vi "Threshold.vi"(8 "error in (no error)":errorcluster, 10 "Threshold":dbl, 11 "DAQ AI in":refnum<class "DAQ AI.lvclass">) -> (0 "error out":errorcluster, 3 "DAQ AI out":refnum<class "DAQ AI.lvclass">)   [LabVIEW 2020, in "DAQ AI.lvlib" / "DAQ AI.lvclass"]
uses:
  DAQ AI.lvclass
  DAQ AI.lvclass/DAQ AI.ctl
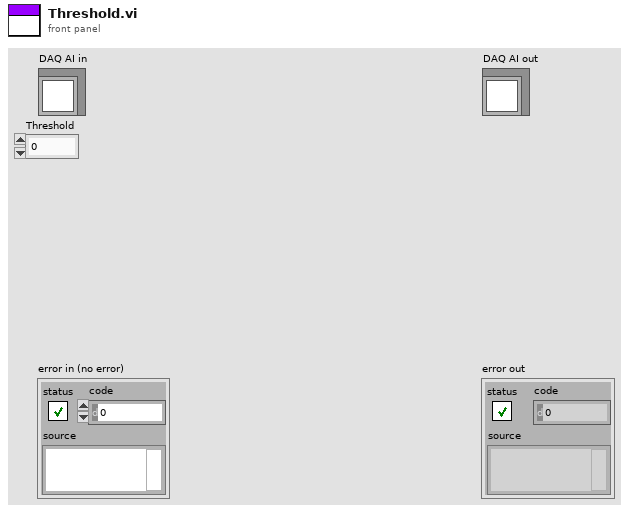
[diagram p1: front panel]
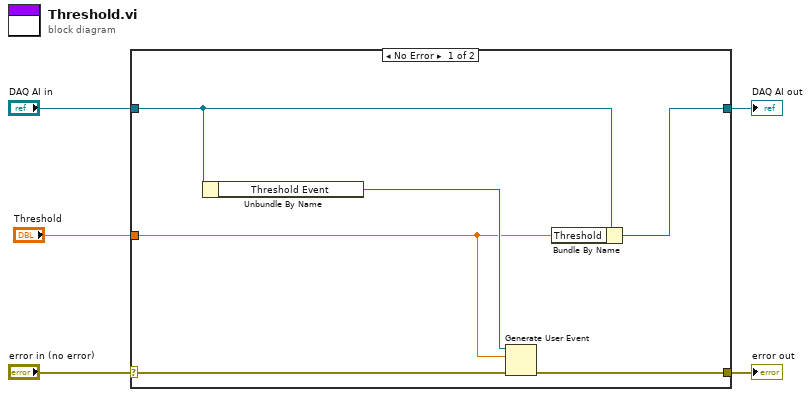
[diagram p0: block diagram]
diagram:
  n1 = case shown="No Error" "error in (no error)" {
    selector: "error in (no error)" -> [w7 w13]
    tunnel: [w6 w13] -> w4
    tunnel: [w10 w12] -> w2
    tunnel: "DAQ AI in" -> [w11 w12]
    tunnel: "Threshold" -> [w8 _]
    frame No Error {
      n2 = Unbundle By Name(w11) -> ("Threshold Event"=w9:refnum<user-event>)
      n3 = Generate User Event(user event=w9, event data cluster=w8, error in=w7) -> (error out=w6:errorcluster)  [unwired: 1 in, 1 out]
      n4 = Bundle By Name(cluster=w11, "Threshold"=w8) -> (w10:refnum<class "DAQ AI.lvclass">)
    }
    frame Error {
    }
  }
  "error out" <- w4
  "DAQ AI out" <- w2
